vi "cmd tester.vi"() -> ()   [LabVIEW 2021]
panel:
  out "return code":i32
  out "standard error":string
  out "standard output":string
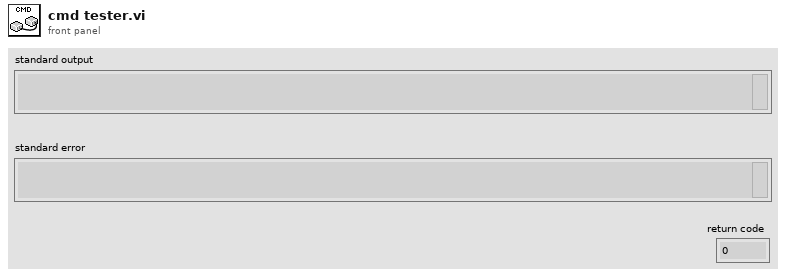
[diagram p1: front panel]
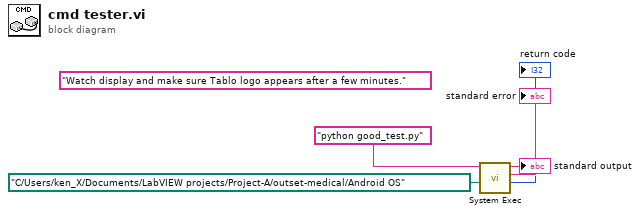
[diagram p0: block diagram]
diagram:
  (unwired) "Watch display and make sure Tablo logo appears after a few minutes."
  n1 = call <vilib>:"System Exec.vi"("working directory"=path "C:/Users/ken_X/Documents/LabVIEW projects/Project-A/outset-medical/Android OS", "command line"="python good_test.py") -> ("return code"=→"return code":i32, "standard error"=→"standard error":string, "standard output"=→"standard output":string)  [unwired: 6 in, 1 out]
